vi "Position GPS Status LED.vi"(8 "error in (no error)":errorcluster, 11 "Button Ref":refnum<vi>) -> (0 "error out":errorcluster)   [LabVIEW 2014]
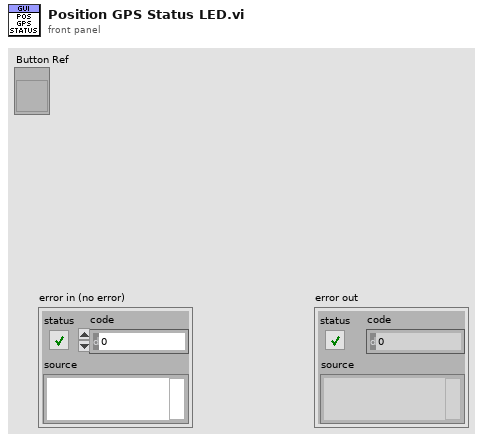
[diagram p1: front panel]
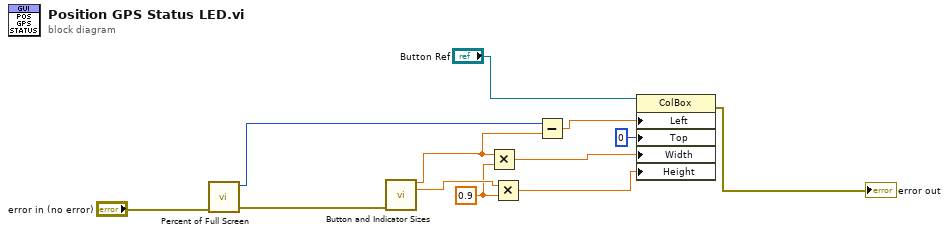
[diagram p0: block diagram]
diagram:
  w7 = 0.9 ("y")
  n1 = call "Percent of Full Screen.vi"("error in (no error)"="error in (no error)") -> ("error out"=w3:errorcluster, "Right"=w4:i16)  [unwired: 8 in, 1 out]
  n2 = call "Button and Indicator Sizes.vi"("error in (no error)"=w3) -> ("Button Width"=w6:dbl, "Button Height"=w10:dbl)  [unwired: 10 in, 3 out]
  n3 = Multiply(x=w6, y=w7) -> (x*y=w8:dbl)
  n4 = Multiply(x=w10, y=w7) -> (x*y=w9:dbl)
  n5 = Subtract(x=w4, y=w6) -> (x-y=w5:dbl)
  n6 = property class="ColBox"(reference="Button Ref", "Left"=w5, "Top"=0 ("Position:Top"), "Width"=w8, "Height"=w9) -> (error out=→"error out":errorcluster)  [unwired: 1 in, 1 out]
